vi "onPlay.vi"(8 "error in (no error)":errorcluster, 10 "Player In":refnum<class "Player.lvclass">, 11 "LockedState in":refnum<class "LockedState.lvclass">) -> (0 "error out":errorcluster, 1 "String":string, 2 "Player Out":refnum<class "Player.lvclass">, 3 "LockedState out":refnum<class "LockedState.lvclass">)   [LabVIEW 2018, in "LockedState.lvclass"]
uses:
  LockedState.lvclass
  Player Class/Player.lvclass
  ReadyState Class/ReadyState.lvclass
  C:/Users/fflores/Documents/LabVIEW-Open-Projects/LabIVEW OOP Design Patterns/State Pattern/State Class/State.lvclass
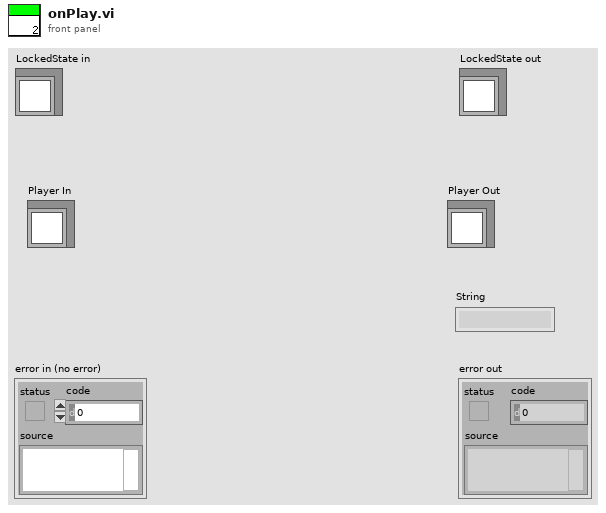
[diagram p1: front panel]
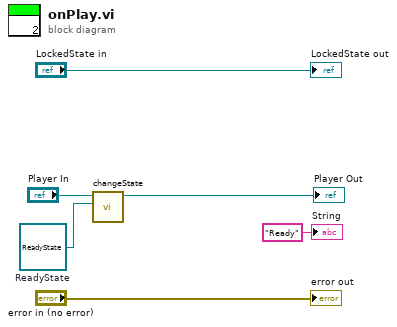
[diagram p0: block diagram]
diagram:
  w3 = refnum<class "ReadyState.lvclass"> refnum  # ReadyState
  n1 = call-dynamic "changeState.vi"("State"=w3, "Player in"="Player In") -> ("Player out"=→"Player Out":refnum<class "Player.lvclass">)  [unwired: 8 in, 1 out]
  "error out" <- "error in (no error)"
  "LockedState out" <- "LockedState in"
  "String" <- "Ready" ("String")
